vi "Data View Display.vi"(8 "error in (no error)":errorcluster, 10 "Name":string, 11 "[V] Main UI in":refnum<class "[V] Main UI.lvclass">) -> (0 "error out":errorcluster, 3 "[V] Main UI out":refnum<class "[V] Main UI.lvclass">)   [LabVIEW 2020, in "[V] Main UI.lvlib" / "[V] Main UI.lvclass"]
uses:
  [V] Main UI.lvclass
  Depden On/MVVM Framework/MVVM Abstruct View/MVVM Abstruct View/MVVM Abstruct View.lvclass/MVVM Abstruct View.ctl
  <vilib>/ActorFramework/Message Enqueuer/Message Enqueuer.lvclass/Message Enqueuer.ctl
  Depden On/MVVM Framework/MVVM Abstruct View/MVVM Abstruct View/Accessor/Read Self-Views.vi
  <vilib>/ActorFramework/Message Enqueuer/Enqueue.vi
  Depden On/Abstruct View/Abstruct View Messages/Insert Panel Msg/Insert Panel Msg.lvclass
  C:/Program Files (x86)/National Instruments/LabVIEW 2020/vi.lib/ActorFramework/Message/Message.lvclass
  <vilib>/ActorFramework/Message Priority Queue/Priority Enqueue.vi
  Depden On/ActorMap/ActorMap.lvclass
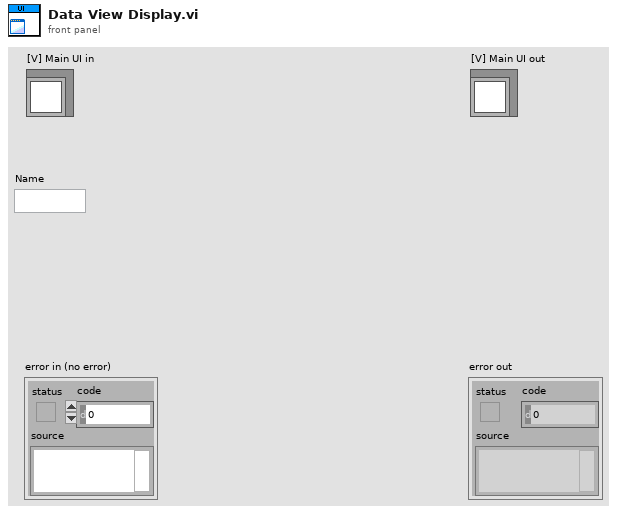
[diagram p1: front panel]
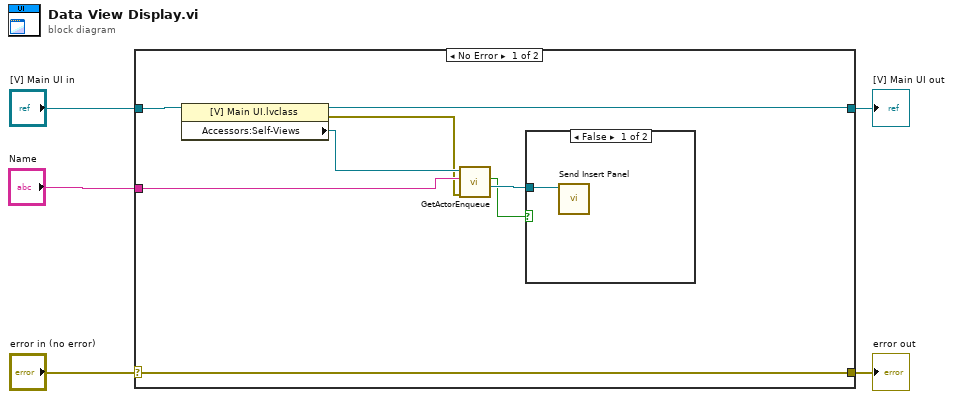
[diagram p0: block diagram]
diagram:
  n1 = case shown="No Error" "error in (no error)" {
    selector: "error in (no error)" -> [w13 w16]
    tunnel: [w13 w16] -> w4
    tunnel: [w7 w15] -> w2
    tunnel: "[V] Main UI in" -> [w9 w15]
    tunnel: "Name" -> [w12 _]
    frame No Error {
      n2 = property class="[V] Main UI.lvclass"(reference=w9) -> (reference out=w7:refnum<class "[V] Main UI.lvclass">, error out=w6:errorcluster, "Accessors:Self-Views"=w8:refnum<class "ActorMap.lvclass">)  [unwired: 1 in]
      n3 = call "GetActorEnqueue.vi"("error in (no error)"=w6, "name"=w12, "ActorMap in"=w8) -> ("Enqueue"=w11:refnum<class "Message Enqueuer.lvclass">, "key not found?"=w10:bool)  [unwired: 5 in, 2 out]
      n4 = case shown="False" w10 {
        tunnel: w11 -> [w14 _]
        frame False {
          n5 = call "Send Insert Panel.vi"("Message Enqueuer"=w14) -> ()  [unwired: 9 in, 2 out]
        }
        frame True {
        }
      }
    }
    frame Error {
    }
  }
  "error out" <- w4
  "[V] Main UI out" <- w2
